vi "CheckTachError.vi"(8 "error in (no error)":errorcluster, 10 "timeout":bool, 11 "fpga vi reference in":refnum<k20>) -> (0 "error out":errorcluster, 3 "fpga vi reference out":refnum<k20>)   [LabVIEW 2017, in "cRIOWfmLib.lvlib"]
uses:
  <vilib>/addons/InsightCM/Devices/Shared/Cms/cRIOWfmAcq/cRIOWfmLib.lvlib
  <vilib>/rvi/errors/niLvFpgaAdjustHostInterfaceError.vi
  <vilib>/rvi/interface/nirviReadWriteControl/nirviReadWriteControl.xnode
  NiFpgaLv.dll
  <vilib>/rvi/interface/Simulation/niFpgaSimulationCallBeginRW.vi
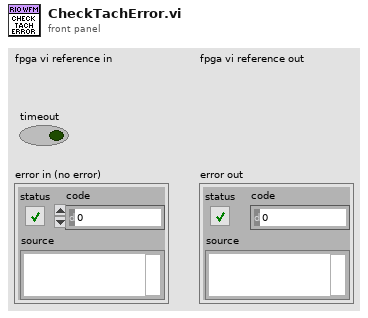
[diagram p1: front panel]
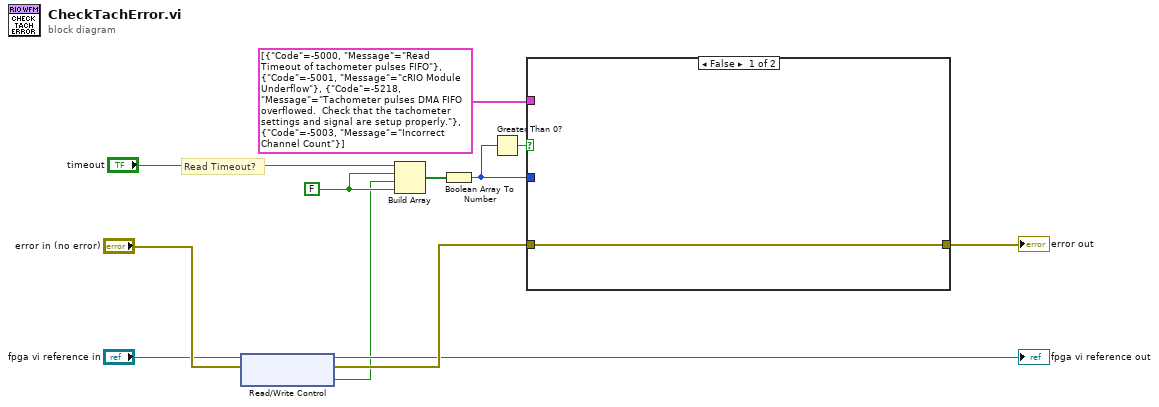
[diagram p0: block diagram]
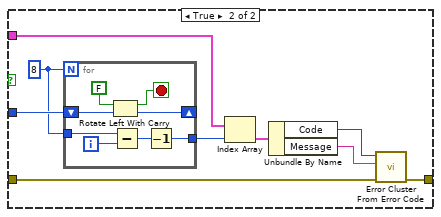
[diagram p2: hidden frame]
diagram:
  w10 = FALSE
  # "Read Timeout?"
  n1 = xnode "Read/Write Control"("FPGA VI Reference In"="fpga vi reference in", "error in"="error in (no error)") -> ("FPGA VI Reference Out"=→"fpga vi reference out":refnum<k20>, "error out"=w12:errorcluster, "Tach FIFO Full"=w3:bool)
  n2 = Build Array("timeout", w10, w3, w10) -> (w4:bool[])
  n3 = Boolean Array To Number(Boolean array=w4) -> (number=w5:u8)
  n4 = Greater Than 0?(x=w5) -> (x > 0?=w6:bool)
  n5 = case shown="False" w6 {
    tunnel: w5 -> [_ w22]
    tunnel: cluster{"Code":i32, "Message":string}[] [{"Code"=-5000, "Message"="Read Timeout of tachometer pulses FIFO"}, {"Code"=-5001, "Message"="cRIO Module Underflow"}, {"Code"=-5218, "Message"="Tachometer pulses DMA FIFO overflowed.  Check that the tachometer settings and signal are setup properly."}, {"Code"=-5003, "Message"="Incorrect Channel Count"}] -> [_ w19]
    tunnel: w12 -> [w13 w15]
    tunnel: [w13 w14] -> w1
    frame False {
    }
    frame True {
      w20 = 8
      n6 = for {
        N: w20 -> [_]
        tunnel: [w24] -> w21
        tunnel: w20 -> [w27]
        shift-right: [w23] -> _
        shift-left: w22 -> [w30]
        i -> [w26]
        stop <- w29 stop-if-true
        n7 = Rotate Left With Carry(2:w30, 3:FALSE ("carry")) -> (0:w23:u8, 1:w29:bool)
        n8 = Subtract(x=w27, y=w26) -> (x-y=w25:i32)
        n9 = Decrement(x=w25) -> (x-1=w24:i32)
      }
      n10 = Index Array(array=w19, index=w21) -> (element=w18:cluster{"Code":i32, "Message":string})
      n11 = Unbundle By Name(w18) -> ("Code"=w17:i32, "Message"=w16:string)
      n12 = call <vilib>:"Error Cluster From Error Code.vi"("error in (no error)"=w15, "error message (\"\")"=w16, "error code (0)"=w17) -> ("error out"=w14:errorcluster)  [unwired: 1 in, 5 out]
    }
  }
  "error out" <- w1
